vi "Configure Modulation.vi"   [LabVIEW 2015, in "SDG X Series.lvlib"]
doc: "Allows users to configure different modulation settings on the function generator.\n\nNote: Modulation is not available if the carrier waveform is DC or Noise."
uses:
  <instrlib>/SDG X Series/SDG X Series.lvlib
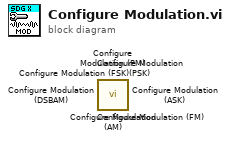
[diagram p0: block diagram]
diagram:
  n1 = call <instrlib>:"Configure Modulation (AM).vi"() -> ()  [unwired: 10 in, 2 out]
  n2 = call <instrlib>:"Configure Modulation (PSK).vi"() -> ()  [unwired: 10 in, 2 out]
  n3 = call <instrlib>:"Configure Modulation (DSBAM).vi"() -> ()  [unwired: 10 in, 2 out]
  n4 = call <instrlib>:"Configure Modulation (ASK).vi"() -> ()  [unwired: 10 in, 2 out]
  n5 = call <instrlib>:"Configure Modulation (FSK).vi"() -> ()  [unwired: 10 in, 2 out]
  n6 = call <instrlib>:"Configure Modulation (PM).vi"() -> ()  [unwired: 10 in, 2 out]
  n7 = call <instrlib>:"Configure Modulation (FM).vi"() -> ()  [unwired: 10 in, 2 out]
